vi "Return Timeout Error.vi"(7 "error source vi name":string, 8 "error in (no error)":errorcluster, 10 "expected iteration":u64=1, 11 "Transfer Group in":refnum<class "Transfer Group.lvclass">) -> (0 "error out":errorcluster, 3 "Transfer Group out":refnum<class "Transfer Group.lvclass">)   [LabVIEW 2017, in "DSF Core.lvlib" / "Transfer Group.lvclass"]
uses:
  Transfer Group.lvclass
  Errors.ctl
  Transfer Group.lvclass/Transfer Group.ctl
  VIs/Constants/Engine Library Name.vi
  <vilib>/NI/Memory Manager/VIs/New Error Cluster Constant (512B).vi
  <vilib>/NI/Memory Manager/VIs/Source.Write.Scalar.Base10 (I32).vi
  <vilib>/NI/Memory Manager/VIs/Source.Write.Scalar.Base10 (U64).vi
  DSF Core.lvlib
  <vilib>/NI/Memory Manager/Static Error Handling.lvlib
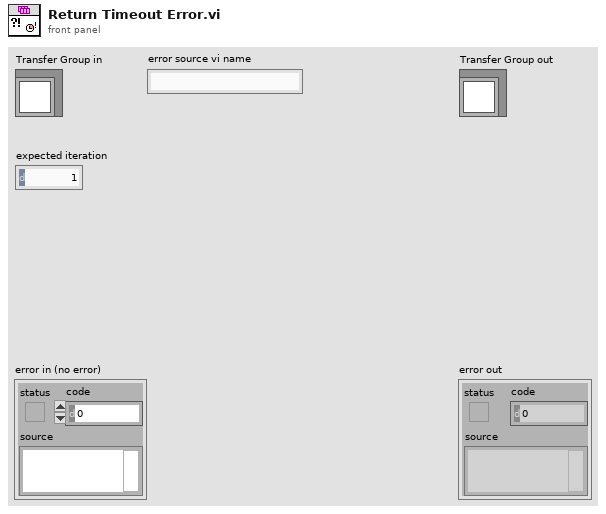
[diagram p1: front panel]
types:
  T1 = typedef "DSF Core.lvlib/Transfer Group.lvclass/Errors.ctl" = enum16{"Return Timeout", "Invalid Iteration"}
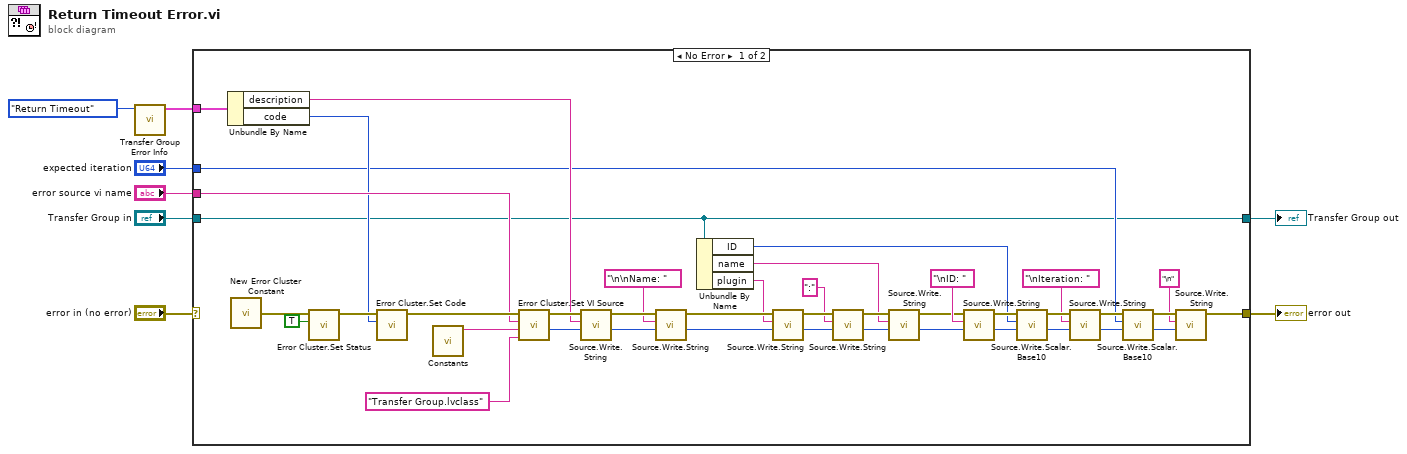
[diagram p0: block diagram]
diagram:
  n1 = call "Transfer Group Error Info.vi"("errors"=Errors."Return Timeout") -> ("error info"=w1:cluster{"code":i32, "description":string})  [unwired: 10 in]
  n2 = case shown="No Error" "error in (no error)" {
    selector: "error in (no error)" -> [_ w50]
    tunnel: [w37 w50] -> w7
    tunnel: [w18 w51] -> w6
    tunnel: "Transfer Group in" -> [w18 w51]
    tunnel: "error source vi name" -> [w41 _]
    tunnel: "expected iteration" -> [w25 _]
    tunnel: w1 -> [w33 _]
    frame No Error {
      n3 = Unbundle By Name(w33) -> ("description"=w28:string, "code"=w32:i32)
      n4 = call-poly <vilib>:"New Error Cluster Constant.vi"() -> ("error out"=w49:errorcluster)  [unwired: 1 in]
      n5 = call <vilib>:"Error Cluster.Set Status.vi"("status (T)"=TRUE, "error in"=w49) -> ("error out"=w48:errorcluster)  [unwired: 9 in]
      n6 = call <vilib>:"Error Cluster.Set Code.vi"("code"=w32, "error in"=w48) -> ("error out"=w47:errorcluster)  [unwired: 9 in]
      n7 = call-poly "Constants.vi"() -> ("Engine Library Name"=w46:string)  [unwired: 11 in]
      n8 = call <vilib>:"Error Cluster.Set VI Source.vi"("class name (\"\")"="Transfer Group.lvclass" ("Engine Library Name"), "library name (\"\")"=w46, "vi name"=w41, "error in"=w47) -> ("new offset"=w30:i32, "error out"=w31:errorcluster)  [unwired: 6 in]
      n9 = call <vilib>:"Source.Write.String.vi"("offset"=w30, "string"=w28, "error in"=w31) -> ("new offset"=w20:i32, "error out"=w21:errorcluster)  [unwired: 7 in]
      n10 = call <vilib>:"Source.Write.String.vi"("offset"=w20, "string"="\n\nName: ", "error in"=w21) -> ("new offset"=w16:i32, "error out"=w17:errorcluster)  [unwired: 7 in]
      n11 = Unbundle By Name(w18) -> ("ID"=w24:i32, "name"=w11:string, "plugin"=w15:string)
      n12 = call <vilib>:"Source.Write.String.vi"("offset"=w16, "string"=w15, "error in"=w17) -> ("new offset"=w14:i32, "error out"=w10:errorcluster)  [unwired: 7 in]
      n13 = call <vilib>:"Source.Write.String.vi"("offset"=w14, "string"=":", "error in"=w10) -> ("new offset"=w12:i32, "error out"=w13:errorcluster)  [unwired: 7 in]
      n14 = call <vilib>:"Source.Write.String.vi"("offset"=w12, "string"=w11, "error in"=w13) -> ("new offset"=w23:i32, "error out"=w22:errorcluster)  [unwired: 7 in]
      n15 = call <vilib>:"Source.Write.String.vi"("offset"=w23, "string"="\nID: ", "error in"=w22) -> ("new offset"=w44:i32, "error out"=w45:errorcluster)  [unwired: 7 in]
      n16 = call-poly <vilib>:"Source.Write.Scalar.Base10.vi"("offset"=w44, "value"=w24, "error in"=w45) -> ("new offset"=w42:i32, "error out"=w43:errorcluster)  [unwired: 7 in]
      n17 = call <vilib>:"Source.Write.String.vi"("offset"=w42, "string"="\nIteration: ", "error in"=w43) -> ("new offset"=w39:i32, "error out"=w40:errorcluster)  [unwired: 7 in]
      n18 = call-poly <vilib>:"Source.Write.Scalar.Base10.vi"("offset"=w39, "value"=w25, "error in"=w40) -> ("new offset"=w36:i32, "error out"=w38:errorcluster)  [unwired: 7 in]
      n19 = call <vilib>:"Source.Write.String.vi"("offset"=w36, "string"="\n", "error in"=w38) -> ("error out"=w37:errorcluster)  [unwired: 7 in, 1 out]
    }
    frame Error {
      # "Incoming error. Pass through."
    }
  }
  "error out" <- w7
  "Transfer Group out" <- w6
